vi "ServoController_clear.vi"(8 "Error In":errorcluster, 11 "Servo Controller Index":u8) -> (0 "Error Out":errorcluster)   [LabVIEW 2013]
uses:
  <vilib>/myRIO/Instrument Drivers/Onboard IO/I2C/vis/Smart Open.vi
  <vilib>/myRIO/Instrument Drivers/Onboard IO/I2C/vis/Configure.vi
  <vilib>/myRIO/Instrument Drivers/Onboard IO/I2C/vis/Write.vi
  <vilib>/myRIO/Instrument Drivers/Onboard IO/I2C/vis/Open.vi
  <vilib>/myRIO/Common/Instrument Driver Framework/myRIO v1.0/I2C/vis/myRIO v1.1 Open I2C.vi
  <vilib>/myRIO/Common/Instrument Driver Framework/Utilities/vis/Validate Channels.vi
  <vilib>/myRIO/Common/Instrument Driver Framework/myRIO v1.0/I2C/vis/myRIO v1.0 Reserve I2C.vi
  <vilib>/myRIO/Common/Instrument Driver Framework/myRIO v1.0/I2C/vis/myRIO v1.0 Build MUX Configuration I2C.vi
  <vilib>/myRIO/Common/Instrument Driver Framework/myRIO v1.0/Resource Manager/vis/myRIO v1.0 Reserve Channel List.vi
  <vilib>/myRIO/Common/Instrument Driver Framework/myRIO v1.0/Resource Manager/vis/myRIO v1.0 Create Configuration List.vi
  <vilib>/myRIO/Common/Instrument Driver Framework/myRIO v1.0/Resource Manager/vis/myRIO v1.0 Reserve Channel.vi
  <vilib>/myRIO/Common/Instrument Driver Framework/myRIO v1.0/Resource Manager/vis/myRIO v1.0 Unreserve Channel.vi
  <vilib>/myRIO/Common/Instrument Driver Framework/myRIO v1.0/Resource Manager/vis/myRIO v1.0 Build Mutex Name.vi
  <vilib>/myRIO/Common/Instrument Driver Framework/myRIO v1.0/myRIO v1.1 Open.vi
  <vilib>/Utility/VariantDataType/GetNumericInfo.vi
  <vilib>/Utility/error.llb/Error Cluster From Error Code.vi
  <vilib>/myRIO/Common/Instrument Driver Framework/Utilities/vis/IO Manager.vi
  <vilib>/myRIO/Common/Instrument Driver Framework/Utilities/vis/Configuration Manager.vi
  <vilib>/myRIO/Common/Instrument Driver Framework/myRIO v1.0/Resource Manager/vis/myRIO v1.0 Configure IO.vi
  <vilib>/myRIO/Common/Instrument Driver Framework/myRIO v1.0/myRIO v1.0 Close.vi
  <vilib>/myRIO/Common/Instrument Driver Framework/myRIO v1.0/I2C/vis/myRIO v1.0 Configure I2C.vi
  <vilib>/myRIO/Common/Instrument Driver Framework/myRIO v1.0/I2C/vis/myRIO v1.0 Write I2C.vi
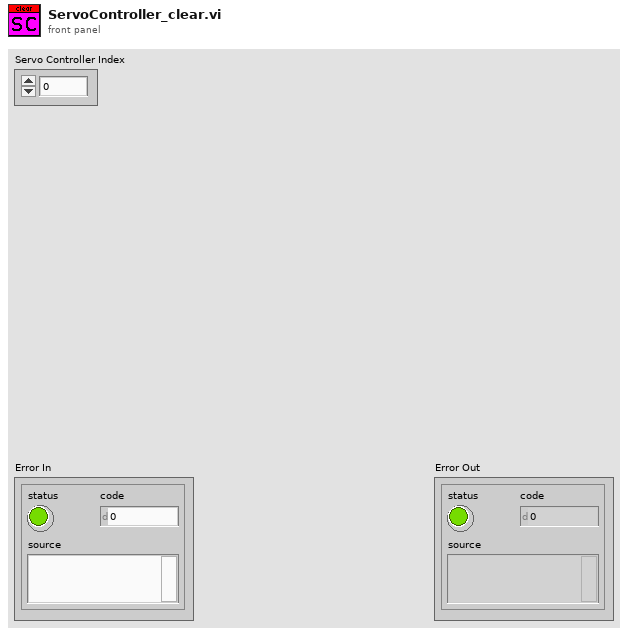
[diagram p1: front panel]
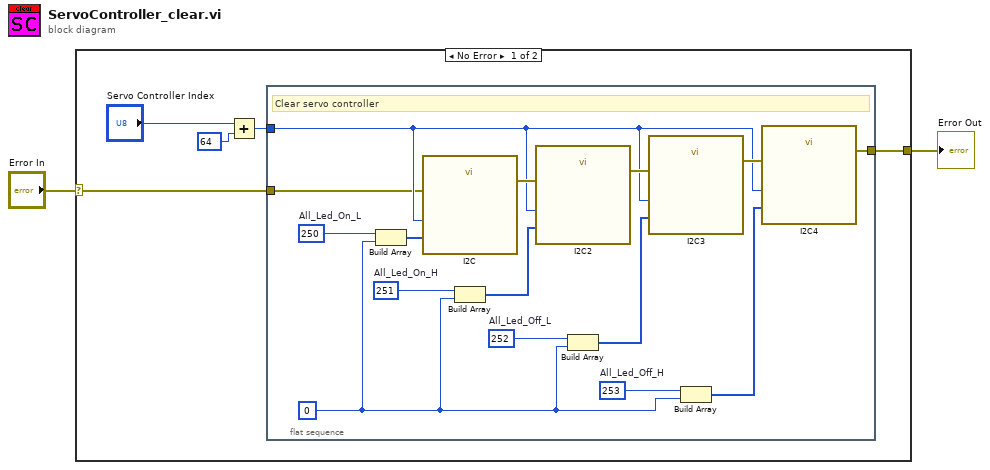
[diagram p0: block diagram]
diagram:
  n1 = case shown="No Error" "Error In" {
    selector: "Error In" -> [w3 w23]
    tunnel: [w5 w23] -> w2
    frame No Error {
      n2 = Add(x="Servo Controller Index", y=u8 64 ("Slave Address (7-bit)")) -> (x+y=w6:u8)
      n3 = flat-sequence {
        tunnel: [w18] -> w5
        tunnel: w6 -> [w17]
        tunnel: w3 -> [w8]
        frame #0 {
          w13 = u8 253  # All_Led_Off_H
          w14 = u8 252  # All_Led_Off_L
          w15 = u8 251  # All_Led_On_H
          w9 = u8 0
          w16 = u8 250  # All_Led_On_L
          # "Clear servo controller"
          n4 = Build Array(w16, w9) -> (w22:u8[])
          n5 = call "I2C"("Slave Address (7-bit)"=w17, "Bytes to Write"=w22, "error in (no error)"=w8) -> ("error out"=w21:errorcluster)  [unwired: 24 in]
          n6 = Build Array(w15, w9) -> (w12:u8[])
          n7 = call "I2C2"("Slave Address (7-bit)"=w17, "Bytes to Write"=w12, "error in (no error)"=w21) -> ("error out"=w20:errorcluster)  [unwired: 24 in]
          n8 = Build Array(w14, w9) -> (w11:u8[])
          n9 = call "I2C3"("Slave Address (7-bit)"=w17, "Bytes to Write"=w11, "error in (no error)"=w20) -> ("error out"=w19:errorcluster)  [unwired: 24 in]
          n10 = Build Array(w13, w9) -> (w10:u8[])
          n11 = call "I2C4"("Slave Address (7-bit)"=w17, "Bytes to Write"=w10, "error in (no error)"=w19) -> ("error out"=w18:errorcluster)  [unwired: 24 in]
        }
      }
    }
    frame Error {
    }
  }
  "Error Out" <- w2
